vi "Limit Switch Control.vi"(11 "Run Mode":T1) -> (0 "Arm Bottom":bool, 1 "Arm Top":bool, 2 "Lift Bottom":bool, 3 "Lift Top":bool)   [LabVIEW 2014]
uses:
  TypeDefs/SRE Enum.ctl
  <vilib>/Rock Robotics/SystemInterfaces/DIO/FPGA_DIOChannel.ctl
  <vilib>/Rock Robotics/WPI/Switch/WPI_SwitchOpenLimit.vi
  Text Variable VIs/Read Number Variable.vi
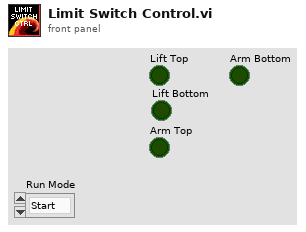
[diagram p1: front panel]
types:
  T1 = typedef "SRE Enum.ctl" = enum16{"Start", "Run", "End"}
  T2 = typedef "FPGA_DIOChannel.ctl" = enum8{"DIO 0", "DIO 1", "DIO 2", "DIO 3", "DIO 4", "DIO 5", "DIO 6", "DIO 7", "DIO 8", "DIO 9", "DIO MXP 0", "DIO MXP 1", "DIO MXP 2", "DIO MXP 3", "DIO MXP 4", "DIO MXP 5", "DIO MXP 6", "DIO MXP 7", "DIO MXP 8", "DIO MXP 9", "DIO MXP 10", "DIO MXP 11", "DIO MXP 12", "DIO MXP 13", "DIO MXP 14", "DIO MXP 15", "Invalid"}
  T3 = typedef "WPI_SwitchDevRef.ctl" = cluster{"DevStatus":errorcluster, "DIO Channel":T2, "Controller":T4, "CntIndex":T5, "Normally Closed":bool}
  T4 = typedef "FPGA_TypedefDigitalModule.ctl" = enum16{"Controller 1"}
  T5 = typedef "FPGA_CounterCtrSystemIndex.ctl" = enum8{"Ctr 0", "Ctr 1", "Ctr 2", "Ctr 3", "Ctr 4", "Ctr 5", "Ctr 6", "Ctr 7", "Invalid"}
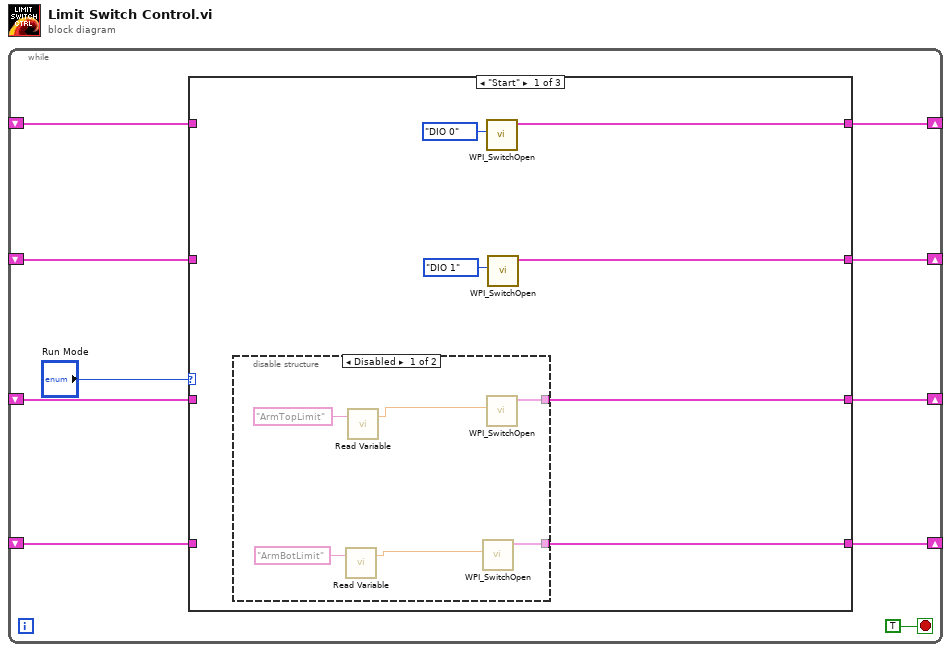
[diagram p0: block diagram]
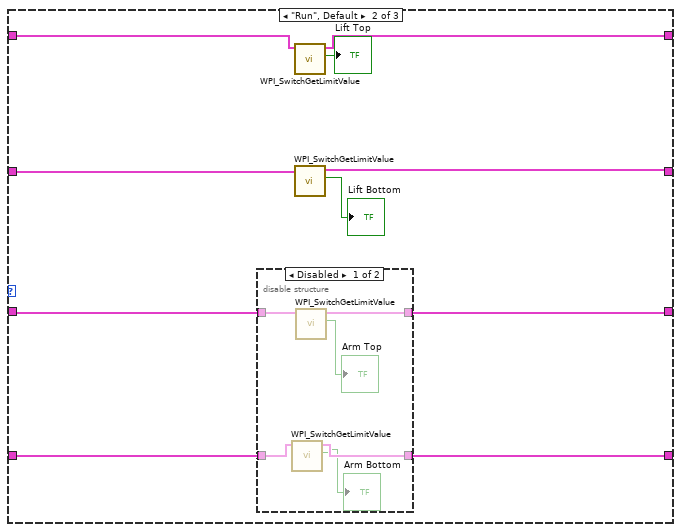
[diagram p3: hidden frame]
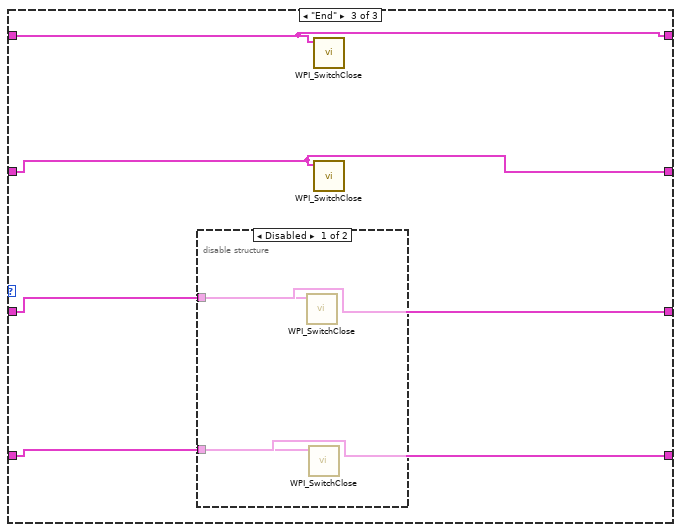
[diagram p5: hidden frame]
diagram:
  n1 = while {
    shift-right: [w7] -> _
    shift-left: _ -> [w4]
    shift-right: [w8] -> _
    shift-left: _ -> [w5]
    shift-right: [w9] -> _
    shift-left: _ -> [w3]
    shift-right: [w6] -> _
    shift-left: _ -> [w2]
    stop <- TRUE stop-if-true
    n2 = case shown="\"Start\"" "Run Mode" {
      tunnel: [w16 w28 w41] -> w9
      tunnel: [w15 w29 w40] -> w8
      tunnel: [w14 w31 w39] -> w7
      tunnel: [w13 w25 w42] -> w6
      tunnel: w5 -> [_ w30 w40]
      tunnel: w4 -> [_ w32 w39]
      tunnel: w3 -> [_ w27 w41]
      tunnel: w2 -> [_ w26 w42]
      frame "Start" {
        n3 = disable-structure shown="Disabled" {
          disable-tunnel: [w22 _] -> w16
          disable-tunnel: [w21 _] -> w13
          frame Disabled {
            n4 = call-poly "Read Variable.vi"("Name"="ArmBotLimit") -> ("number"=w19:dbl)  [unwired: 1 in, 1 out]
            n5 = call-poly "Read Variable.vi"("Name"="ArmTopLimit") -> ("number"=w20:dbl)  [unwired: 1 in, 1 out]
            n6 = call-poly <vilib>:"WPI_SwitchOpen.vi"("DIO Channel"=w19) -> ("SwitchDevRef"=w21:T3)  [unwired: 9 in, 1 out]
            n7 = call-poly <vilib>:"WPI_SwitchOpen.vi"("DIO Channel"=w20) -> ("SwitchDevRef"=w22:T3)  [unwired: 9 in, 1 out]
          }
          frame Enabled {
          }
        }
        n8 = call-poly <vilib>:"WPI_SwitchOpen.vi"("DIO Channel"=FPGA_DIOChannel."DIO 0") -> ("SwitchDevRef"=w14:T3)  [unwired: 9 in, 1 out]
        n9 = call-poly <vilib>:"WPI_SwitchOpen.vi"("DIO Channel"=FPGA_DIOChannel."DIO 1") -> ("SwitchDevRef"=w15:T3)  [unwired: 9 in, 1 out]
      }
      frame "Run", Default {
        n10 = disable-structure shown="Disabled" {
          disable-tunnel: [w38 _] -> w28
          disable-tunnel: w27 -> [w37 _]
          disable-tunnel: w26 -> [w36 _]
          disable-tunnel: [w35 _] -> w25
          frame Disabled {
            n11 = call <vilib>:"WPI_SwitchGetLimitValue.vi"("SwitchDevRef"=w36) -> ("Switch Pressed"=→"Arm Bottom":bool, "SwitchDevRef"=w35:T3)  [unwired: 8 in, 1 out]
            n12 = call <vilib>:"WPI_SwitchGetLimitValue.vi"("SwitchDevRef"=w37) -> ("Switch Pressed"=→"Arm Top":bool, "SwitchDevRef"=w38:T3)  [unwired: 8 in, 1 out]
          }
          frame Enabled {
          }
        }
        n13 = call <vilib>:"WPI_SwitchGetLimitValue.vi"("SwitchDevRef"=w32) -> ("Switch Pressed"=→"Lift Top":bool, "SwitchDevRef"=w31:T3)  [unwired: 8 in, 1 out]
        n14 = call <vilib>:"WPI_SwitchGetLimitValue.vi"("SwitchDevRef"=w30) -> ("Switch Pressed"=→"Lift Bottom":bool, "SwitchDevRef"=w29:T3)  [unwired: 8 in, 1 out]
      }
      frame "End" {
        n15 = disable-structure shown="Disabled" {
          disable-tunnel: w42 -> [w44 _]
          disable-tunnel: w41 -> [w43 _]
          frame Disabled {
            n16 = call <vilib>:"WPI_SwitchClose.vi"("SwitchDevRef"=w43) -> ()  [unwired: 10 in, 1 out]
            n17 = call <vilib>:"WPI_SwitchClose.vi"("SwitchDevRef"=w44) -> ()  [unwired: 10 in, 1 out]
          }
          frame Enabled {
          }
        }
        n18 = call <vilib>:"WPI_SwitchClose.vi"("SwitchDevRef"=w39) -> ()  [unwired: 10 in, 1 out]
        n19 = call <vilib>:"WPI_SwitchClose.vi"("SwitchDevRef"=w40) -> ()  [unwired: 10 in, 1 out]
      }
    }
  }
